vi "test.reqwest_post.vi"() -> ()   [LabVIEW 2020]
uses:
  reqwest/reQwestClient.lvclass
panel:
  out "send body":string
  out "send command":string
  in  "File":path
  in  "error in":errorcluster
  out "response_body":string
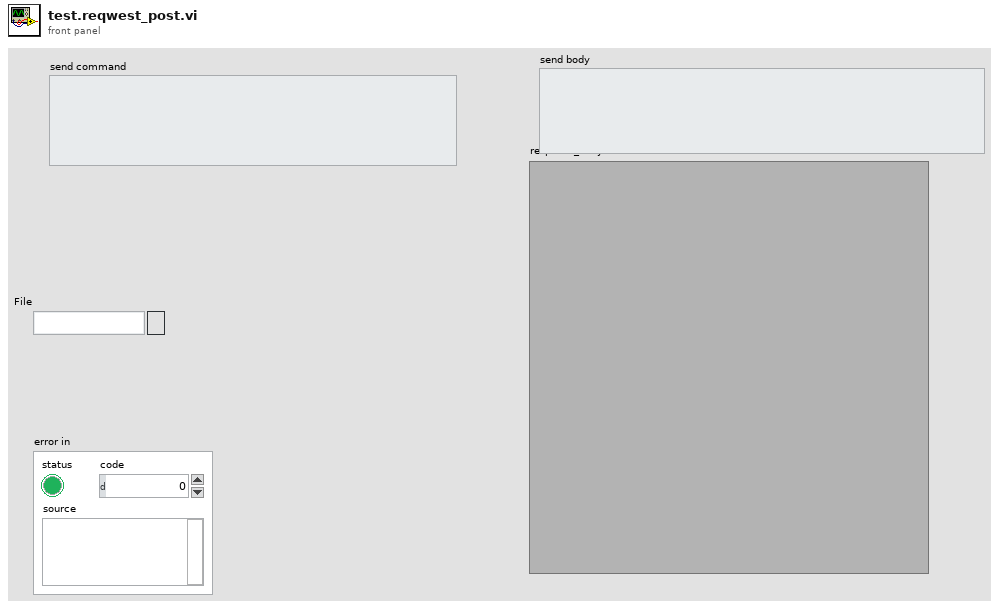
[diagram p1: front panel]
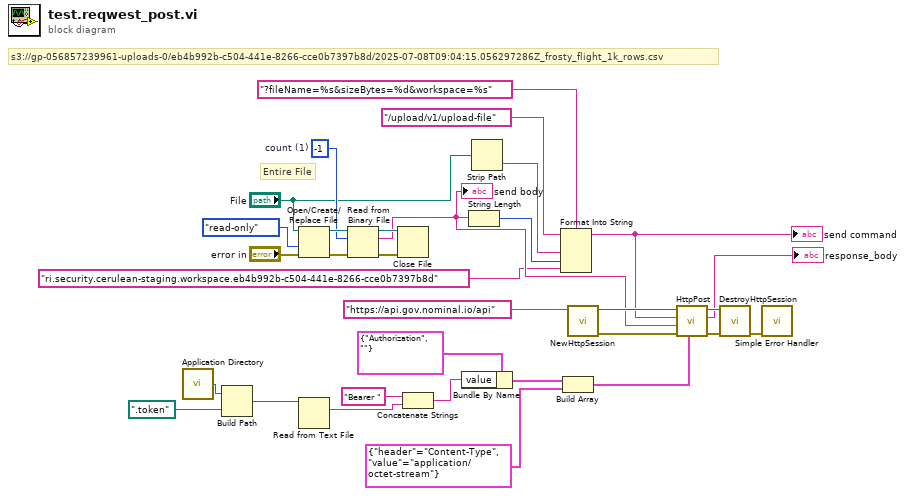
[diagram p0: block diagram]
diagram:
  w10 = -1  # count (1)
  # "s3://gp-056857239961-uploads-0/eb4b992b-c504-441e-8266-cce0b7397b8d/2025-07-08T09:04:15.056297286Z_frosty_flight_1k_rows.csv"
  # "Entire File"
  n1 = call <vilib>:"Application Directory.vi"() -> ("Application Directory"=w27:path)
  n2 = Build Path(base path=w27, name or relative path=path ".token") -> (appended path=w25:path)
  n3 = Open/Create/Replace File(file path (use dialog)="File", error in="error in", access (0:read/write)=enum16{"read/write", "read-only", "write-only"}."read-only") -> (refnum out=w15:refnum<file>, error out=w14:errorcluster)  [unwired: 3 in, 1 out]
  n4 = Read from Text File(file (use dialog)=w25) -> (text=w24:string)  [unwired: 3 in, 3 out]
  n5 = Read from Binary File(8:w14, 10:w10, 11:w15) -> (0:w12:errorcluster, 2:w4:string, 3:w13:refnum<file>)  [unwired: 3 in, 1 out]
  "send body" <- w4
  n6 = Close File(refnum=w13, error in=w12) -> ()  [unwired: 2 out]
  n7 = Concatenate Strings("Bearer " ("value"), w24) -> (w30:string)
  n8 = Bundle By Name(cluster=cluster{"header":string, "value":string} {"header"="Authorization", "value"=""} ("Header"), "value"=w30) -> (w29:cluster{"header":string, "value":string})
  n9 = String Length(string=w4) -> (length=w9:i32)
  n10 = Strip Path(path="File") -> (name=w7:string)  [unwired: 1 out]
  n11 = Format Into String(format string="?fileName=%s&sizeBytes=%d&workspace=%s" ("Path"), initial string="/upload/v1/upload-file" ("Path"), w7, w9, "ri.security.cerulean-staging.workspace.eb4b992b-c504-441e-8266-cce0b7397b8d" ("input 3")) -> (resulting string=w5:string)  [unwired: 1 in, 1 out]
  "send command" <- w5
  n12 = Build Array(w29, cluster{"header":string, "value":string} {"header"="Content-Type", "value"="application/octet-stream"} ("Header")) -> (w17:cluster{"header":string, "value":string}[])
  n13 = call "NewHttpSession.vi"("base url"="https://api.gov.nominal.io/api") -> ("error out"=w20:errorcluster, "reQwestClient"=w21:refnum<class "reQwestClient.lvclass">)  [unwired: 9 in]
  n14 = call "HttpPost.vi"("request specific headers"=w17, "error in"=w20, "body"=w4, "url"=w5, "reQwestClient in"=w21) -> ("error out"=w19:errorcluster, "response_body"=→"response_body":string, "reQwestClient out"=w18:refnum<class "reQwestClient.lvclass">)  [unwired: 4 in]
  n15 = call "DestroyHttpSession.vi"("error in"=w19, "reQwestClient in"=w18) -> ("error out"=w22:errorcluster)  [unwired: 9 in]
  n16 = call <vilib>:"Simple Error Handler.vi"("error in (no error)"=w22) -> ()  [unwired: 4 in, 5 out]
